vi "Set Function Attributes.vi"(10 "Frequency (f)":dbl, 11 "Display State Attributes in":variant) -> (2 "name":string, 3 "Display State Attributes out":variant)   [LabVIEW 2017, in "Test Signal Configuration.xctl"]
uses:
  <vilib>/addons/_XControls/Function Generator Configuration/Test Signal Configuration.xctl
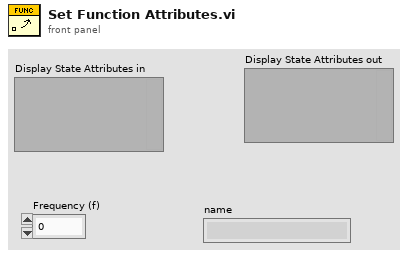
[diagram p1: front panel]
types:
  T1 = typedef "Test Signal Configuration.xctl/signal type.ctl" = enum32{"None", "Tone", "Multitone", "Discrete Sweep", "Continuous Sweep", "Noise"}
  T2 = cluster{"Signal":cluster{"Sample Rate":cluster{"name":string, "default":dbl}, "Signal Type":cluster{"name":string, "signal type":T1}, "Amplitude":cluster{"name":string, "default":dbl}, "Offset":cluster{"name":string, "default":dbl}}, "Function":cluster{"Info":cluster{"name":string, "default":variant}, "Type":cluster{"name":string, "default":u16}, "Frequency":cluster{"name":string, "default":dbl}, "Phase":cluster{"name":string, "default":dbl}}, "Continuous Sweep":cluster{"Info":cluster{"name":string, "default":variant}, "Start":cluster{"name":string, "default":dbl}, "Stop":cluster{"name":string, "default":dbl}, "Duration":cluster{"name":string, "default":dbl}, "Profile":cluster{"name":string, "default":enum16{"Linear", "Logarithmic"}}}, "Discrete Sweep":cluster{"Info":cluster{"name":string, "default":variant}, "Start":cluster{"name":string, "default":dbl}, "Stop":cluster{"name":string, "default":dbl}, "Cycles":cluster{"name":string, "default":dbl}, "Time":cluster{"name":string, "default":dbl}, "Spacing":cluster{"name":string, "default":enum16{"Linear", "Logarithmic"}}, "Steps":cluster{"name":string, "default":i32}}, "Multitone":cluster{"Info":cluster{"name":string, "multitone info":cluster{"frequency":dbl, "amplitude":dbl, "phase":dbl}[]}}, "Noise":cluster{"Info":cluster{"name":string, "default":variant}, "Type":cluster{"name":string, "default":u16}, "Amplitude PDF":cluster{"name":string, "default":enum16{"Gaussian", "Rectangular", "Triangular"}}, "Level":cluster{"name":string, "default":dbl}, "Seed":cluster{"name":string, "default":i32}}, "Configuration":cluster{"Min Frequency":cluster{"name":string, "default":dbl}, "Max Frequency":cluster{"name":string, "default":dbl}, "Max Amplitude":cluster{"name":string, "default":dbl}}}
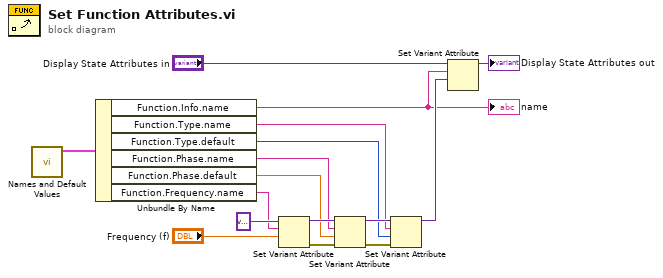
[diagram p0: block diagram]
diagram:
  n1 = call <vilib>:"Names and Default Values.vi"() -> ("Names and Default Values"=w14:T2)  [unwired: 11 in]
  n2 = Unbundle By Name(w14) -> ("Function.Info.name"=w1:string, "Function.Type.name"=w7:string, "Function.Type.default"=w6:u16, "Function.Phase.name"=w8:string, "Function.Phase.default"=w5:dbl, "Function.Frequency.name"=w13:string)
  "name" <- w1
  n3 = Set Variant Attribute(Variant=variant ("Display State Attributes in"), name=w13, value="Frequency (f)") -> (Variant out=w11:variant, error out=w12:errorcluster)  [unwired: 1 in, 1 out]
  n4 = Set Variant Attribute(Variant=w11, name=w8, value=w5, error in=w12) -> (Variant out=w9:variant, error out=w10:errorcluster)  [unwired: 1 out]
  n5 = Set Variant Attribute(Variant=w9, name=w7, value=w6, error in=w10) -> (Variant out=w2:variant)  [unwired: 2 out]
  n6 = Set Variant Attribute(Variant="Display State Attributes in", name=w1, value=w2) -> (Variant out=→"Display State Attributes out":variant)  [unwired: 1 in, 2 out]
